vi "R45_1-FPGA.vi"() -> ()   [LabVIEW 2016]
uses:
  Faraday Cup Readback.ctl
  Aperture Readback.ctl
  Gate Valve Readback.ctl
  Glassman Readback.ctl
  Glassman Control.ctl
  <vilib>/LabVIEW Targets/FPGA/cRIO/shared/nicrio_ModuleControls/nicrio_cRIO-9871_BaudRateEnum.ctl
  <vilib>/LabVIEW Targets/FPGA/cRIO/shared/nicrio_ModuleControls/nicrio_cRIO-9871_ParityEnum.ctl
  <vilib>/LabVIEW Targets/FPGA/cRIO/shared/nicrio_ModuleControls/nicrio_cRIO-9871_StopBitsEnum.ctl
  <vilib>/LabVIEW Targets/FPGA/cRIO/shared/nicrio_ModuleControls/nicrio_cRIO-9871_DataBitsEnum.ctl
  <vilib>/Platform/TimedLoop/XDataNode/timing_clust.ctl
  <vilib>/Platform/TimedLoop/XDataNode/nitl_modes.ctl
  <vilib>/Platform/TimedLoop/XDataNode/wakeup.ctl
  <vilib>/rvi/FXPMathLib/basic elements/FxpIntAccumulator/subVIs/nifxpmath_IntAccumulator_SimConfig.ctl
  <vilib>/rvi/Emulation/niFpgaGetClockAttributes.vi
  <vilib>/rvi/Emulation/niFpgaSctlEmulationGetInTimedLoop.vi
  <vilib>/rvi/Emulation/niFpgaEmulationReportErrorSimple.vi
  <vilib>/rvi/eio/common/nirviEmuTemplateMethod_errors.vi
  <vilib>/rvi/Emulation/niFpgaCriticalErrorInLSC.vi
  <vilib>/rvi/Analysis/common/codeGenErrors/XNode/niFpgaXNodeCodeGenErrorHandle.vi
  <vilib>/rvi/FXPMathLib/basic elements/FxpIntAccumulator/simVIs/DllFxpIntAccumulator_sub.vi
  <vilib>/rvi/eio/common/nirviEmuTemplatePropertySet_errors.vi
  <vilib>/eio/EIONode/EIONode.xnode
  <vilib>/rvi/Analysis/measure/dc-rms/XNode/niFpgaDC-RMS.xnode
  <vilib>/Platform/TimedLoop/XDataNode/XDataNode.xnode
  <vilib>/rvi/FXPMathLib/basic elements/FxpIntAccumulator/XNode/nifxpmath_IntAccumulator.xnode
  <vilib>/rvi/FXPMathLib/FxpMul/XNode/nifxpmath_Multiplier.xnode
  <vilib>/eio/EIOPropertyNode/EIOPropertyNode.xnode
  <vilib>/eio/EIOMethodNode/EIOMethodNode.xnode
  <vilib>/Platform/TimedLoop/XDataNode/XDNodeRunTimeDep.lvlib
  <vilib>/rvi/FXPMathLib/sim/FxpSim.dll
  <vilib>/rvi/eio/common/nirviEmuTemplatePropertyGet_errors.vi
  <vilib>/rvi/eio/common/nirviEmuTemplatePropertyGet_noerrors.vi
  <vilib>/rvi/eio/common/nirviEmuTemplatePropertySet_noerrors.vi
panel:
  out "2nd stage temp":u8[](array[numeric])
  out "Time since repurge":u8[](array[numeric])
  out "Cryo pump error":errorcluster
  out "Cryo 1st stage temp":u8[](array[numeric])
  out "Cryo On-time":u8[](array[numeric])
  out "Cryo status":u8[](array[numeric])
  in  "RT error":bool
  in  "Switch Mag Aperture actuator":bool
  in  "Switch Mag FC actuator":bool
  out "Cup-Aperture Control Loop Error":errorcluster
  out "Vac Cluster 1 Ion Gauge 2":u8[](array[numeric])
  out "Vac Cluster 1 Convectron 2":u8[](array[numeric])
  out "Vac Cluster 1 Convectron 1":u8[](array[numeric])
  out "Vac Cluster 1 Ion Gauge 1":u8[](array[numeric])
  out "Vacuum Gauge 1 error":errorcluster
  in  "Right Steerer Voltage set":T1
  in  "Down Steerer Voltage set":T1
  out "HV Control error":errorcluster
  in  "Up Steerer Voltage set":T1
  in  "Left Steerer Voltage set":T1
  out "Right Steerer readback":T2
  out "Left Steerer readback":T2
  out "Down Steerer readback":T2
  out "Up Steerer readback":T2
  out "HV readback error":errorcluster
  out "Position-Sensor readback error":errorcluster
  out "Cryo Pump GV position":T3
  out "Beamline GV 1 position":T3
  out "Switch Mag Aperture Position":T4
  out "Switch Mag FC Position":T5
  out "Vac and GV interlock error":errorcluster
  in  "Vac cluster 2 Ion Gauge Interlock":bool=TRUE
  out "Vac cluster 1 Convectron Guage Interlock":bool
  out "Vac cluster 1 Ion Guage Interlock":bool
  in  "Beamline GV 1 actuator":bool
  in  "Cryo GV actuator":bool
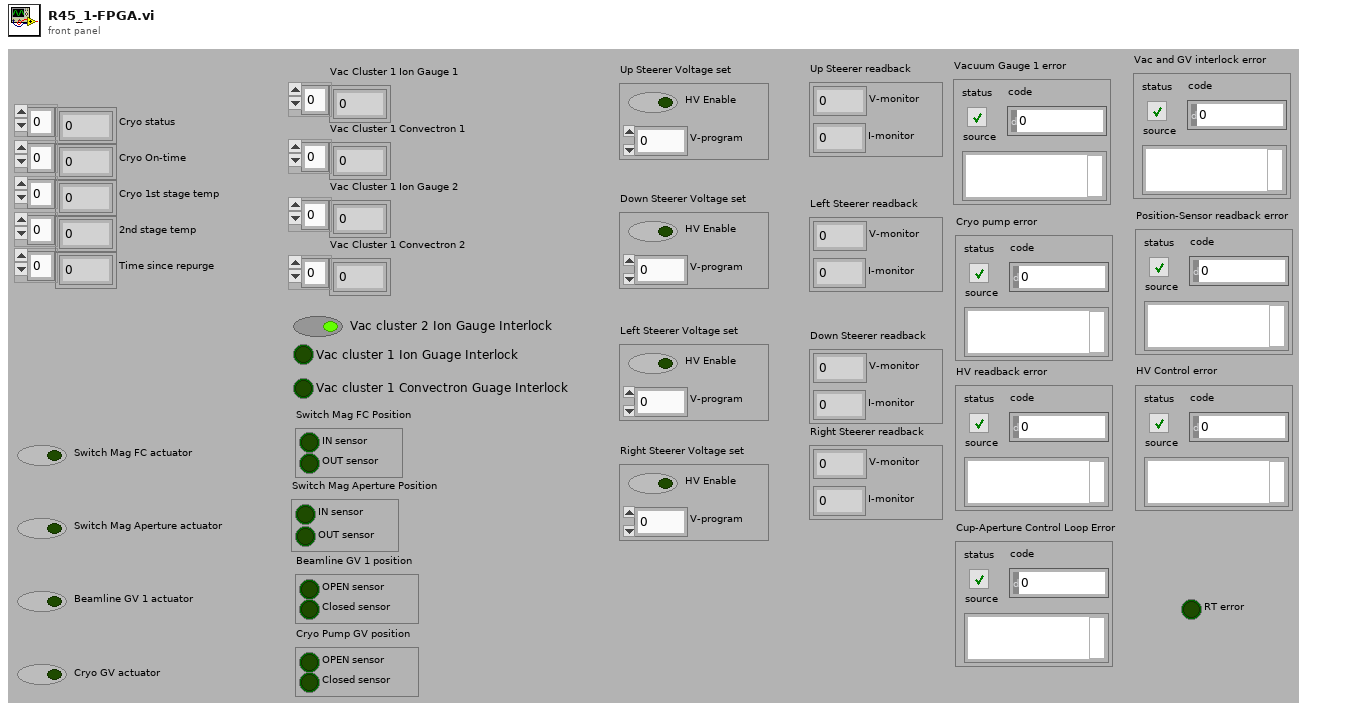
[diagram p1: front panel]
types:
  T1 = typedef "Glassman Control.ctl" = cluster{"V-program":fxp<+/-,20,7>, "HV Enable":bool}
  T2 = typedef "Glassman Readback.ctl" = cluster{"I-monitor":fxp<+/-,26,5>, "V-monitor":fxp<+/-,26,7>}
  T3 = typedef "Gate Valve Readback.ctl" = cluster{"OPEN sensor":bool, "Closed sensor":bool}
  T4 = typedef "Aperture Readback.ctl" = cluster{"IN sensor":bool, "OUT sensor":bool}
  T5 = typedef "Faraday Cup Readback.ctl" = cluster{"IN sensor":bool, "OUT sensor":bool}
  T6 = typedef "nicrio_cRIO-9871_ParityEnum.ctl" = enum8{"None", "Odd", "Even", "Mark", "Space"}
  T7 = typedef "nicrio_cRIO-9871_StopBitsEnum.ctl" = enum8{"1", "1.5", "2"}
  T8 = typedef "nicrio_cRIO-9871_DataBitsEnum.ctl" = enum8{"5", "6", "7", "8"}
  T9 = typedef "nicrio_cRIO-9871_BaudRateEnum.ctl" = enum16{"75 bps", "110 bps", "134 bps", "150 bps", "300 bps", "600 bps", "1200 bps", "1800 bps", "2400 bps", "4800 bps", "7200 bps", "9600 bps", "14.4 kbps", "19.2 kbps", "28.8 kbps", "38.4 kbps", "57.6 kbps", "115.2 kbps", "230.4 kbps", "460.8 kbps", "921.6 kbps"}
  T10 = typedef "XDNodeRunTimeDep.lvlib/timing_clust.ctl" = cluster{"Expected End [f-1]":u64, "Actual End [f-1]":u64, "Finished Late? [f-1]":bool, "Expected End [i-1]":u64, "Actual End [i-1]":u64, "Finished Late? [i-1]":bool, "Expected Start [i]":u64, "Actual Start [i]":u64, "Expected Start [f]":u64, "Actual Start [f]":u64, "Source Name":string, "Structure Name":string, "Period":i64, "Deadline":i64, "Offset":i64, "Start":i64, "Priority":i32, "Timeout":i32, "Mode":T11, "Wakeup Reason":T12, "Error":errorcluster, "Source Type":string, "Secondary Source Type":string, "Global End Time":u64, "Global Start Time":u64, "Frame Duration":u64, "Iteration Duration":u64, "Assigned CPU":i32, "I/O Scan Engine Mode":u32}
  T11 = typedef "XDNodeRunTimeDep.lvlib/nitl_modes.ctl" = enum32{"No Change", "Process missed periods, maintain original phase", "Discard missed periods, maintain original phase", "Process missed periods, ignore original phase", "Discard missed periods, ignore original phase"}
  T12 = typedef "XDNodeRunTimeDep.lvlib/wakeup.ctl" = enum32{"Normal", "Aborted", "Asynchronous wakeup", "Timing source error", "Timed loop error", "Timeout"}
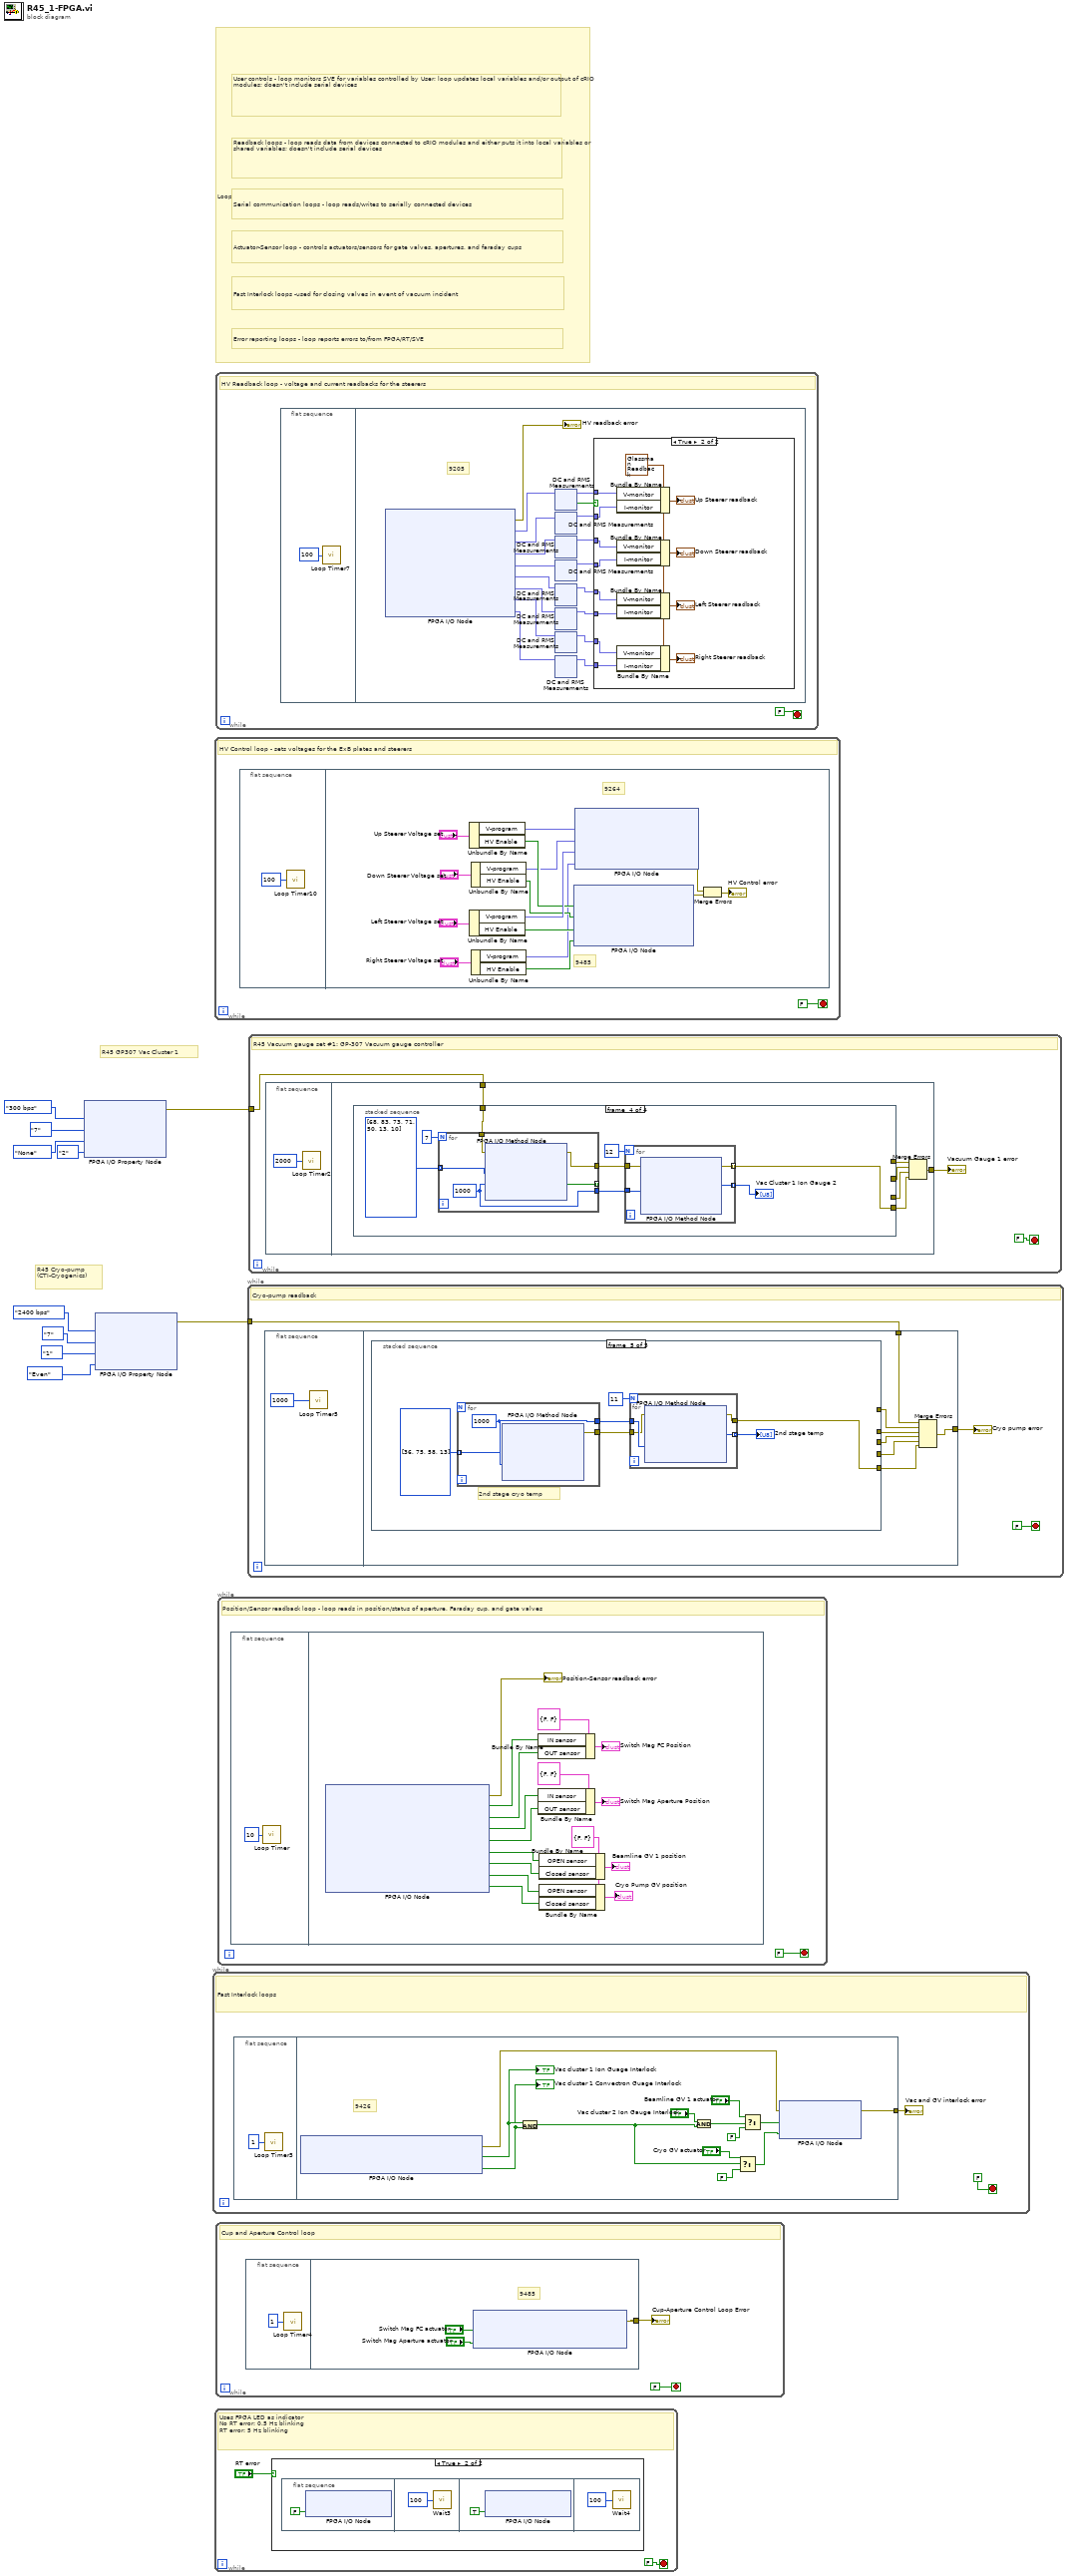
[diagram p0: block diagram]
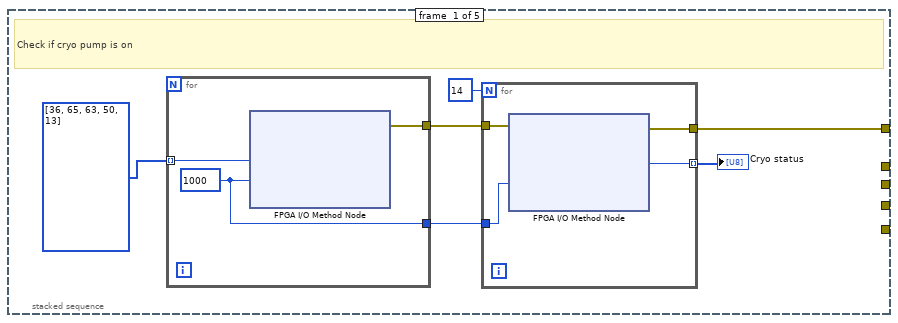
[diagram p2: hidden frame]
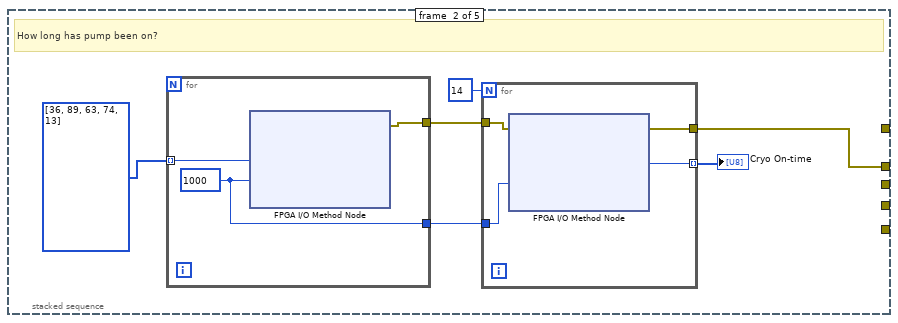
[diagram p3: hidden frame]
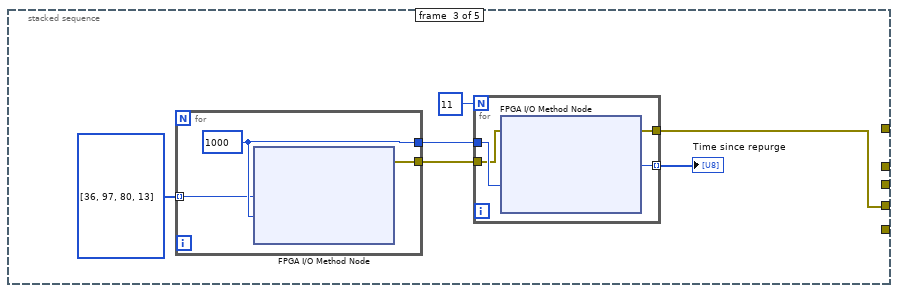
[diagram p4: hidden frame]
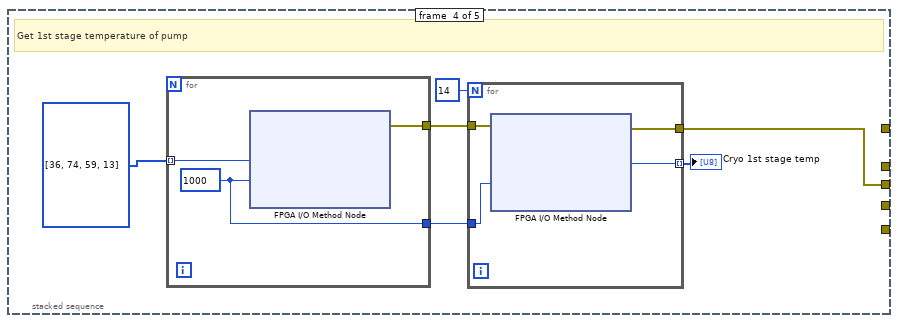
[diagram p5: hidden frame]
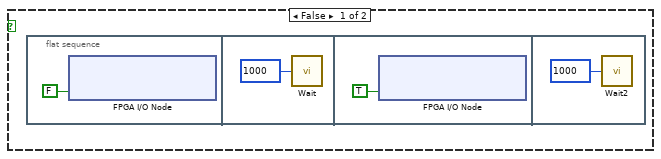
[diagram p6: hidden frame]
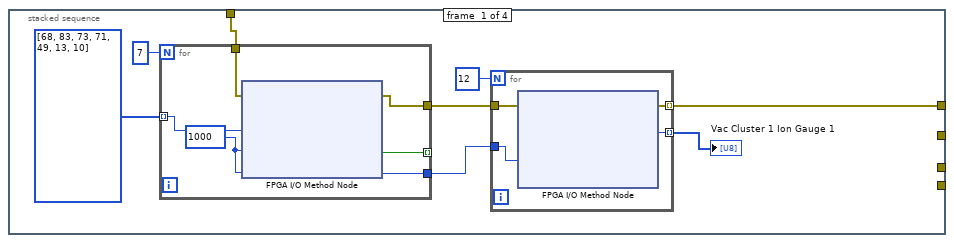
[diagram p7: hidden frame]
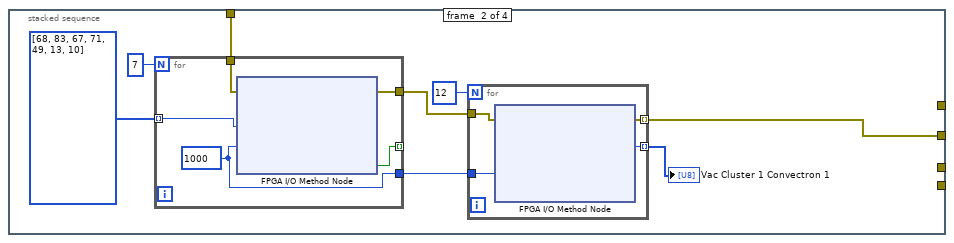
[diagram p8: hidden frame]
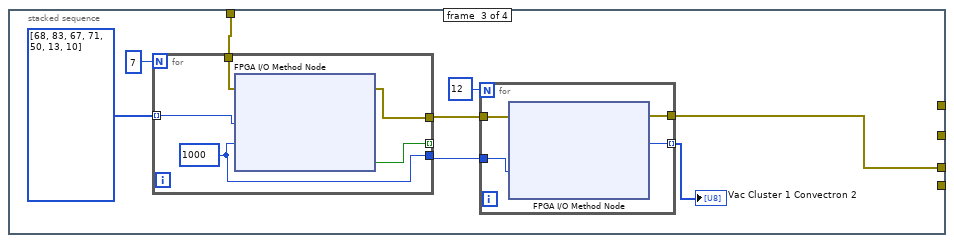
[diagram p9: hidden frame]
diagram:
  # "Actuator-Sensor loop - controls actuators/sensors for gate valves, apertures, and faraday cups"
  # "R45 Cryo-pump\n(CTI-Cryogenics)"
  # "R45 GP307 Vac Cluster 1"
  # "Fast Interlock loops -used for closing valves in event of vacuum incident"
  # "Error reporting loops - loop reports errors to/from FPGA/RT/SVE"
  # "Serial communication loops - loop reads/writes to serially connected devices"
  # "Readback loops - loop reads data from devices connected to cRIO modules and either puts it into local variables or shared variables; doesn't include serial devices"
  # "User controls - loop monitors SVE for variables controlled by User; loop updates local variables and/or output of cRIO modules; doesn't include serial devices"
  # "Loop legend - loops are color coded by responsibility"
  n1 = xnode "FPGA I/O Property Node"("Baud Rate"=nicrio_cRIO-9871_BaudRateEnum."300 bps", "Data Bits"=nicrio_cRIO-9871_DataBitsEnum."7", "Parity"=nicrio_cRIO-9871_ParityEnum."None", "Stop Bits"=nicrio_cRIO-9871_StopBitsEnum."2") -> ("error out"=w6:errorcluster)  [unwired: 2 in, 1 out]
  n2 = xnode "FPGA I/O Property Node"("Baud Rate"=nicrio_cRIO-9871_BaudRateEnum."2400 bps", "Data Bits"=nicrio_cRIO-9871_DataBitsEnum."7", "Stop Bits"=nicrio_cRIO-9871_StopBitsEnum."1", "Parity"=nicrio_cRIO-9871_ParityEnum."Even") -> ("error out"=w1:errorcluster)  [unwired: 2 in, 1 out]
  n3 = while {
    stop <- FALSE stop-if-true
    # "Fast Interlock loops"
    n4 = flat-sequence {
      tunnel: [w14] -> w11
      frame #0 {
        n5 = call "Loop Timer3"("Count(uSec)"=u32 1 ("Count(Ticks)")) -> ()  [unwired: 1 out]
      }
      frame #1 {
        # "9426"
        n6 = xnode "FPGA I/O Node"() -> ("error out"=w15:errorcluster, "Vac cluster 1 Ion Gauge Interlock"=w26:bool, "Vac cluster 1 Convectron Gauge Interlock"=w25:bool)  [unwired: 3 in, 2 out]
        "Vac cluster 1 Ion Guage Interlock" <- w26
        "Vac cluster 1 Convectron Guage Interlock" <- w25
        n7 = And(x=w26, y=w25) -> (x .and. y?=w17:bool)
        n8 = And(x="Vac cluster 2 Ion Gauge Interlock", y=w17) -> (x .and. y?=w18:bool)
        n9 = Select(t="Cryo GV actuator", s=w17, f=FALSE) -> (s? t:f=w24:bool)
        n10 = Select(t="Beamline GV 1 actuator", s=w18, f=FALSE) -> (s? t:f=w20:bool)
        n11 = xnode "FPGA I/O Node"("error in"=w15, "Beamline GV 1"=w20, "Cryo GV"=w24) -> ("error out"=w14:errorcluster)  [unwired: 2 in, 2 out]
      }
    }
    "Vac and GV interlock error" <- w11
  }
  n12 = while {
    stop <- FALSE stop-if-true
    # "HV Control loop - sets voltages for the ExB plates and steerers"
    n13 = flat-sequence {
      frame #0 {
        n14 = call "Loop Timer10"("Count(mSec)"=u32 100 ("Count(Ticks)")) -> ()  [unwired: 1 out]
      }
      frame #1 {
        # "9485"
        # "9264"
        n15 = Unbundle By Name("Up Steerer Voltage set") -> ("V-program"=w41:fxp<+/-,20,7>, "HV Enable"=w39:bool)
        n16 = Unbundle By Name("Left Steerer Voltage set") -> ("V-program"=w40:fxp<+/-,20,7>, "HV Enable"=w38:bool)
        n17 = Unbundle By Name("Down Steerer Voltage set") -> ("V-program"=w32:fxp<+/-,20,7>, "HV Enable"=w31:bool)
        n18 = Unbundle By Name("Right Steerer Voltage set") -> ("V-program"=w30:fxp<+/-,20,7>, "HV Enable"=w29:bool)
        n19 = xnode "FPGA I/O Node"("Up Steerer HV Enable"=w39, "Down Steerer HV Enable"=w31, "Left Steerer HV Enable"=w38, "Right Steerer HV Enable"=w29) -> ("error out"=w35:errorcluster)  [unwired: 5 in, 4 out]
        n20 = xnode "FPGA I/O Node"("Up Steerer Voltage set"=w41, "Down Steerer Voltage set"=w32, "Left Steerer Voltage set"=w40, "Right Steerer Voltage set"=w30) -> ("error out"=w36:errorcluster)  [unwired: 5 in, 4 out]
        n21 = Merge Errors(w36, w35) -> (→"HV Control error":errorcluster)
      }
    }
  }
  n22 = while {
    stop <- FALSE stop-if-true
    # "Uses FPGA LED as indicator\nNo RT error: 0.5 Hz blinking\nRT error: 5 Hz blinking"
    n23 = case shown="True" "RT error" {
      frame False {
        n24 = flat-sequence {
          frame #0 {
            n25 = xnode "FPGA I/O Node"("USER FPGA LED"=FALSE ("FPGA LED")) -> ()  [unwired: 1 in, 1 out]
          }
          frame #1 {
            n26 = call "Wait"("Count(mSec)"=u16 1000) -> ()  [unwired: 1 out]
          }
          frame #2 {
            n27 = xnode "FPGA I/O Node"("USER FPGA LED"=TRUE ("FPGA LED")) -> ()  [unwired: 1 in, 1 out]
          }
          frame #3 {
            n28 = call "Wait2"("Count(mSec)"=u16 1000) -> ()  [unwired: 1 out]
          }
        }
      }
      frame True {
        n29 = flat-sequence {
          frame #0 {
            n30 = xnode "FPGA I/O Node"("USER FPGA LED"=FALSE ("FPGA LED")) -> ()  [unwired: 1 in, 1 out]
          }
          frame #1 {
            n31 = call "Wait3"("Count(mSec)"=u16 100) -> ()  [unwired: 1 out]
          }
          frame #2 {
            n32 = xnode "FPGA I/O Node"("USER FPGA LED"=TRUE ("FPGA LED")) -> ()  [unwired: 1 in, 1 out]
          }
          frame #3 {
            n33 = call "Wait4"("Count(mSec)"=u16 100) -> ()  [unwired: 1 out]
          }
        }
      }
    }
  }
  n34 = while {
    stop <- FALSE stop-if-true
    # "HV Readback loop - voltage and current readbacks for the steerers"
    n35 = flat-sequence {
      frame #0 {
        n36 = call "Loop Timer7"("Count(mSec)"=u32 100 ("Count(Ticks)")) -> ()  [unwired: 1 out]
      }
      frame #1 {
        # "9205"
        n37 = xnode "FPGA I/O Node"() -> ("error out"=→"HV readback error":errorcluster, "Up Steerer Voltage read"=w71:fxp<+/-,26,5>, "Up Steerer Current read"=w69:fxp<+/-,26,5>, "Down Steerer Voltage read"=w68:fxp<+/-,26,5>, "Down Steerer Current read"=w67:fxp<+/-,26,5>, "Left Steerer Voltage read"=w66:fxp<+/-,26,5>, "Left Steerer Current read"=w65:fxp<+/-,26,5>, "Right Steerer Voltage read"=w64:fxp<+/-,26,5>, "Right Steerer Current read"=w63:fxp<+/-,26,5>)  [unwired: 9 in, 8 out]
        n38 = xnode "DC and RMS Measurements"("input data"=w71) -> ("DC"=w73:fxp<+/-,26,5>, "output valid"=w72:bool)  [unwired: 1 in]
        n39 = xnode "DC and RMS Measurements"("input data"=w69) -> ("DC"=w57:fxp<+/-,26,5>)  [unwired: 1 in, 1 out]
        n40 = xnode "DC and RMS Measurements"("input data"=w68) -> ("DC"=w56:fxp<+/-,26,5>)  [unwired: 1 in, 1 out]
        n41 = xnode "DC and RMS Measurements"("input data"=w67) -> ("DC"=w58:fxp<+/-,26,5>)  [unwired: 1 in, 1 out]
        n42 = xnode "DC and RMS Measurements"("input data"=w66) -> ("DC"=w59:fxp<+/-,26,5>)  [unwired: 1 in, 1 out]
        n43 = xnode "DC and RMS Measurements"("input data"=w65) -> ("DC"=w60:fxp<+/-,26,5>)  [unwired: 1 in, 1 out]
        n44 = xnode "DC and RMS Measurements"("input data"=w64) -> ("DC"=w61:fxp<+/-,26,5>)  [unwired: 1 in, 1 out]
        n45 = xnode "DC and RMS Measurements"("input data"=w63) -> ("DC"=w62:fxp<+/-,26,5>)  [unwired: 1 in, 1 out]
        n46 = case shown="True" w72 {
          tunnel: w73 -> [_ w646]
          tunnel: w57 -> [_ w645]
          tunnel: w56 -> [_ w634]
          tunnel: w58 -> [_ w644]
          tunnel: w59 -> [_ w643]
          tunnel: w60 -> [_ w642]
          tunnel: w61 -> [_ w641]
          tunnel: w62 -> [_ w640]
          frame False {
          }
          frame True {
            w635 = T2 {"I-monitor"=0.0, "V-monitor"=0.0} ("Glassman Readback")
            n47 = Bundle By Name(cluster=w635, "V-monitor"=w646, "I-monitor"=w645) -> (→"Up Steerer readback":T2)
            n48 = Bundle By Name(cluster=w635, "V-monitor"=w634, "I-monitor"=w644) -> (→"Down Steerer readback":T2)
            n49 = Bundle By Name(cluster=w635, "V-monitor"=w643, "I-monitor"=w642) -> (→"Left Steerer readback":T2)
            n50 = Bundle By Name(cluster=w635, "V-monitor"=w641, "I-monitor"=w640) -> (→"Right Steerer readback":T2)
          }
        }
      }
    }
  }
  n51 = while {
    stop <- FALSE stop-if-true
    # "Cup and Aperture Control loop"
    n52 = flat-sequence {
      tunnel: [w730] -> w727
      frame #0 {
        n53 = call "Loop Timer4"("Count(mSec)"=u32 1 ("Count(Ticks)")) -> ()  [unwired: 1 out]
      }
      frame #1 {
        # "9485"
        n54 = xnode "FPGA I/O Node"("Switch Magnet FC Actuator"="Switch Mag FC actuator", "Switch Magnet Aperture Actuator"="Switch Mag Aperture actuator") -> ("error out"=w730:errorcluster)  [unwired: 3 in, 2 out]
      }
    }
    "Cup-Aperture Control Loop Error" <- w727
  }
  n55 = while {
    stop <- FALSE stop-if-true
    # "Position/Sensor readback loop - loop reads in position/status of aperture, Faraday cup, and gate valves"
    n56 = flat-sequence {
      frame #0 {
        n57 = call "Loop Timer"("Count(mSec)"=u32 10 ("Count(Ticks)")) -> ()  [unwired: 1 out]
      }
      frame #1 {
        w744 = T3 {"OPEN sensor"=FALSE, "Closed sensor"=FALSE} ("Gate Valve")
        n58 = xnode "FPGA I/O Node"() -> ("error out"=→"Position-Sensor readback error":errorcluster, "Switch Magnet FC IN sensor"=w748:bool, "Switch Magnet FC OUT sensor"=w747:bool, "Switch Magnet Aperture IN sensor"=w746:bool, "Switch Magnet Aperture OUT sensor"=w745:bool, "Beamline GV 1 OPEN sensor"=w743:bool, "Beamline GV 1 CLOSED sensor"=w736:bool, "Cryo Pump GV OPEN sensor"=w742:bool, "Cryo Pump GV CLOSED sensor"=w741:bool)  [unwired: 9 in, 8 out]
        n59 = Bundle By Name(cluster=T5 {"IN sensor"=FALSE, "OUT sensor"=FALSE} ("Faraday Cup"), "IN sensor"=w748, "OUT sensor"=w747) -> (→"Switch Mag FC Position":T5)
        n60 = Bundle By Name(cluster=T4 {"IN sensor"=FALSE, "OUT sensor"=FALSE} ("Aperture"), "IN sensor"=w746, "OUT sensor"=w745) -> (→"Switch Mag Aperture Position":T4)
        n61 = Bundle By Name(cluster=w744, "OPEN sensor"=w743, "Closed sensor"=w736) -> (→"Beamline GV 1 position":T3)
        n62 = Bundle By Name(cluster=w744, "OPEN sensor"=w742, "Closed sensor"=w741) -> (→"Cryo Pump GV position":T3)
      }
    }
  }
  n63 = while {
    tunnel: w1 -> [w752]
    stop <- FALSE stop-if-true
    # "Cryo-pump readback"
    n64 = flat-sequence {
      tunnel: w752 -> [w761]
      tunnel: [w760] -> w751
      frame #0 {
        n65 = call "Loop Timer5"("Count(mSec)"=u32 1000) -> ()  [unwired: 1 out]
      }
      frame #1 {
        n66 = stacked-sequence {
          tunnel: [_ w775 _ _ _] -> w759
          tunnel: [w762 _ _ _ _] -> w758
          tunnel: [_ _ _ w801 _] -> w757
          tunnel: [_ _ w788 _ _] -> w756
          tunnel: [_ _ _ _ w814] -> w755
          frame #0 {
            # "Check if cryo pump is on"
            n67 = for {
              tunnel: u8[] [36, 65, 63, 50, 13] ("unsigned byte array") -> [w774] mode=indexing
              tunnel: [w773] -> w765
              tunnel: [w772] -> w763
              w773 = 1000 ("Timeout (ms)")
              n68 = xnode "FPGA I/O Method Node"("Data"=w774, "Timeout (ms)"=w773) -> ("error out"=w772:errorcluster)  [unwired: 2 in, 2 out]
            }
            n69 = for {
              N: 14 -> [_]
              tunnel: [w771] -> w767 mode=indexing
              tunnel: w765 -> [w770]
              tunnel: w763 -> [w769]
              tunnel: [w768] -> w762
              n70 = xnode "FPGA I/O Method Node"("error in"=w769, "Timeout (ms)"=w770) -> ("error out"=w768:errorcluster, "Data"=w771:u8)  [unwired: 1 in, 2 out]
            }
            "Cryo status" <- w767
          }
          frame #1 {
            # "How long has pump been on?"
            n71 = for {
              tunnel: u8[] [36, 89, 63, 74, 13] ("unsigned byte array") -> [w787] mode=indexing
              tunnel: [w786] -> w778
              tunnel: [w785] -> w776
              w786 = 1000 ("Timeout (ms)")
              n72 = xnode "FPGA I/O Method Node"("Data"=w787, "Timeout (ms)"=w786) -> ("error out"=w785:errorcluster)  [unwired: 2 in, 2 out]
            }
            n73 = for {
              N: 14 -> [_]
              tunnel: [w784] -> w780 mode=indexing
              tunnel: w778 -> [w783]
              tunnel: w776 -> [w782]
              tunnel: [w781] -> w775
              n74 = xnode "FPGA I/O Method Node"("error in"=w782, "Timeout (ms)"=w783) -> ("error out"=w781:errorcluster, "Data"=w784:u8)  [unwired: 1 in, 2 out]
            }
            "Cryo On-time" <- w780
          }
          frame #2 {
            n75 = for {
              tunnel: [w800] -> w793
              tunnel: u8[] [36, 97, 80, 13] ("unsigned byte array") -> [w798] mode=indexing
              tunnel: [w799] -> w789
              w800 = 1000 ("Timeout (ms)")
              n76 = xnode "FPGA I/O Method Node"("Data"=w798, "Timeout (ms)"=w800) -> ("error out"=w799:errorcluster)  [unwired: 2 in, 2 out]
            }
            n77 = for {
              N: 11 -> [_]
              tunnel: w793 -> [w797]
              tunnel: [w796] -> w790 mode=indexing
              tunnel: w789 -> [w795]
              tunnel: [w794] -> w788
              n78 = xnode "FPGA I/O Method Node"("error in"=w795, "Timeout (ms)"=w797) -> ("error out"=w794:errorcluster, "Data"=w796:u8)  [unwired: 1 in, 2 out]
            }
            "Time since repurge" <- w790
          }
          frame #3 {
            # "Get 1st stage temperature of pump"
            n79 = for {
              tunnel: u8[] [36, 74, 59, 13] ("unsigned byte array") -> [w813] mode=indexing
              tunnel: [w812] -> w804
              tunnel: [w811] -> w802
              w812 = 1000 ("Timeout (ms)")
              n80 = xnode "FPGA I/O Method Node"("Data"=w813, "Timeout (ms)"=w812) -> ("error out"=w811:errorcluster)  [unwired: 2 in, 2 out]
            }
            n81 = for {
              N: 14 -> [_]
              tunnel: [w810] -> w806 mode=indexing
              tunnel: w804 -> [w809]
              tunnel: w802 -> [w808]
              tunnel: [w807] -> w801
              n82 = xnode "FPGA I/O Method Node"("error in"=w808, "Timeout (ms)"=w809) -> ("error out"=w807:errorcluster, "Data"=w810:u8)  [unwired: 1 in, 2 out]
            }
            "Cryo 1st stage temp" <- w806
          }
          frame #4 {
            # "2nd stage cryo temp"
            n83 = for {
              tunnel: [w826] -> w819
              tunnel: u8[] [36, 75, 58, 13] ("unsigned byte array") -> [w825] mode=indexing
              tunnel: [w824] -> w815
              w826 = 1000 ("Timeout (ms)")
              n84 = xnode "FPGA I/O Method Node"("Data"=w825, "Timeout (ms)"=w826) -> ("error out"=w824:errorcluster)  [unwired: 2 in, 2 out]
            }
            n85 = for {
              N: 11 -> [_]
              tunnel: w819 -> [w823]
              tunnel: [w822] -> w816 mode=indexing
              tunnel: w815 -> [w821]
              tunnel: [w820] -> w814
              n86 = xnode "FPGA I/O Method Node"("error in"=w821, "Timeout (ms)"=w823) -> ("error out"=w820:errorcluster, "Data"=w822:u8)  [unwired: 1 in, 2 out]
            }
            "2nd stage temp" <- w816
          }
        }
        n87 = Merge Errors(w761, w758, w759, w757, w756, w755) -> (w760:errorcluster)
      }
    }
    "Cryo pump error" <- w751
  }
  n88 = while {
    tunnel: w6 -> [w828]
    stop <- FALSE stop-if-true
    # "R45 Vacuum gauge set #1: GP-307 Vacuum gauge controller"
    n89 = flat-sequence {
      tunnel: w828 -> [w836]
      tunnel: [w831] -> w827
      frame #0 {
        n90 = call "Loop Timer2"("Count(mSec)"=u32 2000 ("Count(Ticks)")) -> ()  [unwired: 1 out]
      }
      frame #1 {
        n91 = stacked-sequence {
          tunnel: [_ _ w873 _] -> w833
          tunnel: [_ _ _ w889] -> w832
          tunnel: w836 -> [w839 w856 w871 w888]
          tunnel: [w837 _ _ _] -> w835
          tunnel: [_ w855 _ _] -> w834
          frame #0 {
            n92 = for {
              N: 7 -> [_]
              tunnel: [w853] -> w840
              tunnel: [w852] -> _ mode=indexing
              tunnel: u8[] [68, 83, 73, 71, 49, 13, 10] ("unsigned byte array") -> [w851] mode=indexing
              tunnel: w839 -> [w850]
              tunnel: [w849] -> w838
              w853 = 1000 ("Timeout (ms)")
              n93 = xnode "FPGA I/O Method Node"("error in"=w850, "Data"=w851, "Timeout (ms)"=w853) -> ("error out"=w849:errorcluster, "Timed Out"=w852:bool)  [unwired: 1 in, 1 out]
            }
            n94 = for {
              N: 12 -> [_]
              tunnel: w840 -> [w848]
              tunnel: [w847] -> w841 mode=indexing
              tunnel: w838 -> [w846]
              tunnel: [w845] -> w837 mode=indexing
              n95 = xnode "FPGA I/O Method Node"("error in"=w846, "Timeout (ms)"=w848) -> ("error out"=w845:errorcluster, "Data"=w847:u8)  [unwired: 1 in, 2 out]
            }
            "Vac Cluster 1 Ion Gauge 1" <- w841
          }
          frame #1 {
            n96 = for {
              N: 7 -> [_]
              tunnel: [w869] -> w861
              tunnel: [w868] -> _ mode=indexing
              tunnel: u8[] [68, 83, 67, 71, 49, 13, 10] ("unsigned byte array") -> [w870] mode=indexing
              tunnel: w856 -> [w867]
              tunnel: [w866] -> w854
              w869 = 1000 ("Timeout (ms)")
              n97 = xnode "FPGA I/O Method Node"("error in"=w867, "Data"=w870, "Timeout (ms)"=w869) -> ("error out"=w866:errorcluster, "Timed Out"=w868:bool)  [unwired: 1 in, 1 out]
            }
            n98 = for {
              N: 12 -> [_]
              tunnel: w861 -> [w865]
              tunnel: [w864] -> w857 mode=indexing
              tunnel: w854 -> [w863]
              tunnel: [w862] -> w855 mode=indexing
              n99 = xnode "FPGA I/O Method Node"("error in"=w863, "Timeout (ms)"=w865) -> ("error out"=w862:errorcluster, "Data"=w864:u8)  [unwired: 1 in, 2 out]
            }
            "Vac Cluster 1 Convectron 1" <- w857
          }
          frame #2 {
            n100 = for {
              N: 7 -> [_]
              tunnel: [w885] -> w878
              tunnel: [w886] -> _ mode=indexing
              tunnel: u8[] [68, 83, 67, 71, 50, 13, 10] ("unsigned byte array") -> [w887] mode=indexing
              tunnel: [w884] -> w874
              tunnel: w871 -> [w883]
              w885 = 1000 ("Timeout (ms)")
              n101 = xnode "FPGA I/O Method Node"("error in"=w883, "Data"=w887, "Timeout (ms)"=w885) -> ("error out"=w884:errorcluster, "Timed Out"=w886:bool)  [unwired: 1 in, 1 out]
            }
            n102 = for {
              N: 12 -> [_]
              tunnel: w878 -> [w882]
              tunnel: [w881] -> w872 mode=indexing
              tunnel: w874 -> [w880]
              tunnel: [w879] -> w873
              n103 = xnode "FPGA I/O Method Node"("error in"=w880, "Timeout (ms)"=w882) -> ("error out"=w879:errorcluster, "Data"=w881:u8)  [unwired: 1 in, 2 out]
            }
            "Vac Cluster 1 Convectron 2" <- w872
          }
          frame #3 {
            n104 = for {
              N: 7 -> [_]
              tunnel: [w902] -> w895
              tunnel: [w904] -> _ mode=indexing
              tunnel: u8[] [68, 83, 73, 71, 50, 13, 10] ("unsigned byte array") -> [w903] mode=indexing
              tunnel: [w901] -> w890
              tunnel: w888 -> [w900]
              w902 = 1000 ("Timeout (ms)")
              n105 = xnode "FPGA I/O Method Node"("error in"=w900, "Data"=w903, "Timeout (ms)"=w902) -> ("error out"=w901:errorcluster, "Timed Out"=w904:bool)  [unwired: 1 in, 1 out]
            }
            n106 = for {
              N: 12 -> [_]
              tunnel: w895 -> [w899]
              tunnel: [w898] -> w891 mode=indexing
              tunnel: w890 -> [w897]
              tunnel: [w896] -> w889 mode=indexing
              n107 = xnode "FPGA I/O Method Node"("error in"=w897, "Timeout (ms)"=w899) -> ("error out"=w896:errorcluster, "Data"=w898:u8)  [unwired: 1 in, 2 out]
            }
            "Vac Cluster 1 Ion Gauge 2" <- w891
          }
        }
        n108 = Merge Errors(w835, w834, w833, w832) -> (w831:errorcluster)
      }
    }
    "Vacuum Gauge 1 error" <- w827
  }
